vi "DefaultFromINI.vi"(8 "error in (no error)":errorcluster, 11 "ChromaAcLoad":refnum<class "ChromaAcLoad.lvclass">) -> (0 "error out":errorcluster, 3 "ChromaAcLoad":refnum<class "ChromaAcLoad.lvclass">)   [LabVIEW 2018, in "AcPwrPlugins.lvlib" / "ChromaAcLoad.lvclass"]
doc: "This VI reads the properties from the INI file and puts them into the LabVIEW class for further use."
uses:
  ChromaAcLoad.lvclass
  F:/Program Files (x86)/National Instruments/LabVIEW 2018/user.lib/NIST/BaseClasses/BasePlugin_class/BasePlugin.lvclass
  F:/Projects/ICDAS/NistPluggableModules/AcPwr/AcPwrPlugins/AcPwrBaseClass/AcPwrBase.lvclass
  TypeDefs/Device(s)Settings.ctl
  TypeDefs/ConfigMode.ctl
  TypeDefs/Measurements.ctl
  TypeDefs/MeasurementType.ctl
  <userlib>/NIST/BaseClasses/BasePlugin_class/BasePlugin.lvclass/BasePlugin.ctl
  <userlib>/NIST/BaseClasses/BasePlugin_class/Accessors/Read PluginIniFilePath.vi
  AcPwrBaseClass/AcPwrBase.lvclass
  <vilib>/Utility/config.llb/NI_LVConfig.lvlib
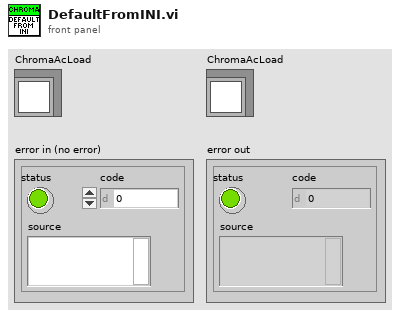
[diagram p1: front panel]
types:
  T1 = typedef "AcPwrPlugins.lvlib/ChromaAcLoad.lvclass/Measurements.ctl" = cluster{"Handle":string, "Name":string, "Enabled":bool, "Measurement Value":dbl, "Hold Peak Current Measurement":bool, "btnMeasFetch":bool, "ProtectionStatusString":string, "Measurement Type":T2}[]
  T2 = typedef "AcPwrPlugins.lvlib/ChromaAcLoad.lvclass/MeasurementType.ctl" = enum16{"Voltage (Vrms or V)", "Current (Arms or A)", "Power (W)", "Peak Voltage (V)", "Peak Current (A)", "Peak Power (W)", "Frequency (Hz)", "Resistance (Ohms)", "Voltage Overshoot (V)", "Positive Peak Current (A)", "Voltage Undershoot (V)", "Negative Peak Current (A)", "Apparent Power (VA)", "Reacitive Power (VAR)", "Voltage THD", "Power Factor", "Current's Crest Factor"}
  T3 = typedef "AcPwrPlugins.lvlib/ChromaAcLoad.lvclass/Device(s)Settings.ctl" = cluster{"Configuration Mode":T4, "Phases":cluster{"Handle":string, "Name":string, "Phase Select":i32, "Instrument Options":string, "id query (T)":bool, "reset device (T)":bool, "Load Short Circuited":bool, "Line Synchronization":bool, "Load Current (A/Arms)":dbl, "Load Voltage (V/Vrms)":dbl, "Load Power (W)":dbl, "Load Resistance (Ohms)":dbl, "Load Current Peak Limit (A)":dbl, "Load Current Limit (A/Arms)":dbl, "Load Power Limit (W)":dbl, "Synch Frequency (Hz)":dbl, "Priority":enum16{"CF Only", "PF Only", "Both (CF)", "Both (PF)"}, "Crest Factor":dbl, "Power Factor":dbl, "Slew Rate":cluster{"Rise Slew Rate (A/ms)":i32, "Fall Slew Rate (A/ms)":i32}, "LC/RLC Mode":cluster{"Capacitance (uF)":i32, "Inductance (uH)":i32, "Series Resistance (Ohm)":dbl, "Parallel Resistance (Ohm)":dbl}, "Timing":cluster{"TimingOn":enum16{""}, "Hours":u32, "Minutes":u32, "Seconds":dbl, "CutoffVoltage":dbl}, "Connected":bool}[], "MeasName":string}
  T4 = typedef "AcPwrPlugins.lvlib/ChromaAcLoad.lvclass/ConfigMode.ctl" = enum16{"Constant Voltage (DC)", "Constant Power (DC)", "Constant Power (AC)", "Constant Current (DC)", "Constant Current (AC)", "Constant Resistance (DC)", "Constant Resistance (AC)", "Rectified Mode (DC)", "Inrush (AC)", "RLC CP (AC)", "RLC (AC)"}
  T5 = typedef "NI_LVConfig.lvlib/Config Data RefNum.ctl" = refnum<k1>
  T6 = typedef "INIInfo.ctl" = cluster{"Module Name":string, "INI File Name":string, "Class Name":string, "INI File Name Without Extension":string, "Module.Class.INI File Name":string, "Visualization VI Path":path, "Instrument Class Path":path}
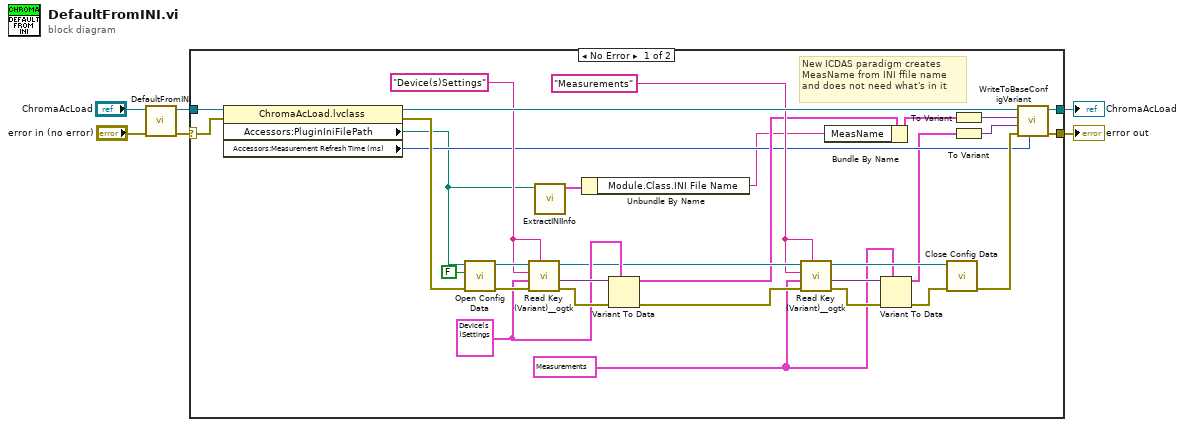
[diagram p0: block diagram]
diagram:
  n1 = call-parent "DefaultFromINI.vi"("error in (no error)"="error in (no error)", "AcPwrBase"="ChromaAcLoad") -> ("error out"=w4:errorcluster, "AcPwrBase"=w3:refnum<class "ChromaAcLoad.lvclass">)  [unwired: 8 in]
  n2 = case shown="No Error" w4 {
    selector: w4 -> [w29 w38]
    tunnel: w3 -> [w37 w39]
    tunnel: [w16 w39] -> w2
    tunnel: [w15 w38] -> w1
    frame No Error {
      w18 = "Measurements" ("section")
      w19 = T1 [{"Handle"="", "Name"="", "Enabled"=FALSE, "Measurement Value"=0.0, "Hold Peak Current Measurement"=FALSE, "btnMeasFetch"=TRUE, "ProtectionStatusString"="", "Measurement Type"=enum."Voltage (Vrms or V)"}] ("Measurements")
      w26 = T3 {"Configuration Mode"=enum."Constant Voltage (DC)", "Phases"=[], "MeasName"=""} ("Device Properties")
      w30 = "Device(s)Settings" ("section")
      # "New ICDAS paradigm creates\nMeasName from INI ffile name\nand does not need what's in it"
      n3 = property class="ChromaAcLoad.lvclass"(reference=w37, error in=w29) -> (reference out=w31:refnum<class "ChromaAcLoad.lvclass">, error out=w28:errorcluster, "Accessors:PluginIniFilePath"=w9:path, "Accessors:Measurement Refresh Time (ms)"=w13:u32)
      n4 = call <vilib>:"Open Config Data.vi"("error in (no error)"=w28, "create file if necessary (T)"=FALSE, "configuration file path"=w9) -> ("error out"=w34:errorcluster, "refnum"=w35:T5)  [unwired: 6 in, 1 out]
      n5 = call <userlib>:"Read Key (Variant)__ogtk.vi"("section"=w30, "error in (no error)"=w34, "type"=w26, "key (optional)"=w30, "refnum"=w35) -> ("error out"=w32:errorcluster, "key-value"=w33:variant, "refnum out"=w23:T5)  [unwired: 3 in, 1 out]
      n6 = call "ExtractINIInfo.vi"("INI File Path"=w9) -> ("INI Info"=w8:T6)  [unwired: 8 in, 2 out]
      n7 = Unbundle By Name(w8) -> ("Module.Class.INI File Name"=w7:string)
      n8 = Variant To Data(error in=w32, type=w26, Variant=w33) -> (data=w14:T3, error out=w20:errorcluster)
      n9 = call <userlib>:"Read Key (Variant)__ogtk.vi"("section"=w18, "error in (no error)"=w20, "type"=w19, "key (optional)"=w18, "refnum"=w23) -> ("error out"=w25:errorcluster, "key-value"=w24:variant, "refnum out"=w22:T5)  [unwired: 3 in, 1 out]
      n10 = Bundle By Name(cluster=w14, "MeasName"=w7) -> (w10:T3)
      n11 = Variant To Data(error in=w25, type=w19, Variant=w24) -> (data=w12:T1, error out=w21:errorcluster)
      n12 = call <vilib>:"Close Config Data.vi"("error in (no error)"=w21, "refnum"=w22) -> ("error out"=w27:errorcluster)  [unwired: 8 in, 1 out]
      n13 = To Variant(anything=w10) -> (Variant=w17:variant)
      n14 = To Variant(anything=w12) -> (Variant=w11:variant)
      n15 = call-dynamic "WriteToBaseConfigVariant.vi"("Measurement Refresh Time (ms)"=w13, "error in (no error)"=w27, "Meas"=w11, "Config"=w17, "ChromaAcLoad in"=w31) -> ("error out"=w15:errorcluster, "ChromaAcLoad out"=w16:refnum<class "ChromaAcLoad.lvclass">)  [unwired: 5 in]
    }
    frame Error {
    }
  }
  "error out" <- w1
  "ChromaAcLoad" <- w2
